vi "init.vi"(8 "error in (no error)":errorcluster, 11 "USD Actor in":refnum<class "USD Actor.lvclass">) -> (0 "error out":errorcluster, 3 "USD Actor out":refnum<class "USD Actor.lvclass">)   [LabVIEW 2020, in "USD Actor.lvlib" / "USD Actor.lvclass"]
uses:
  USD Actor.lvclass
  USD Actor.lvclass/USD Actor.ctl
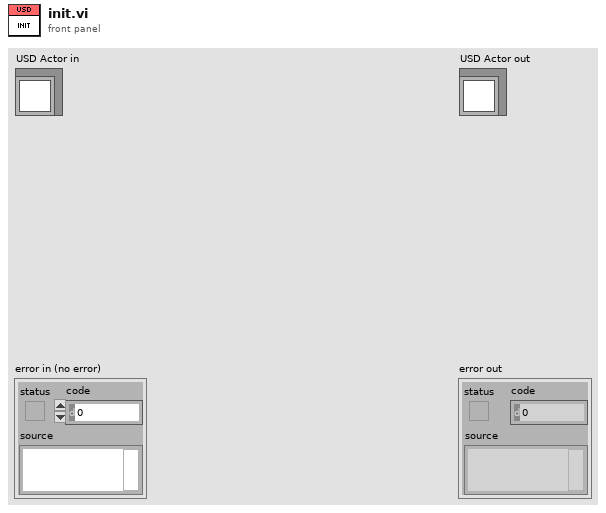
[diagram p1: front panel]
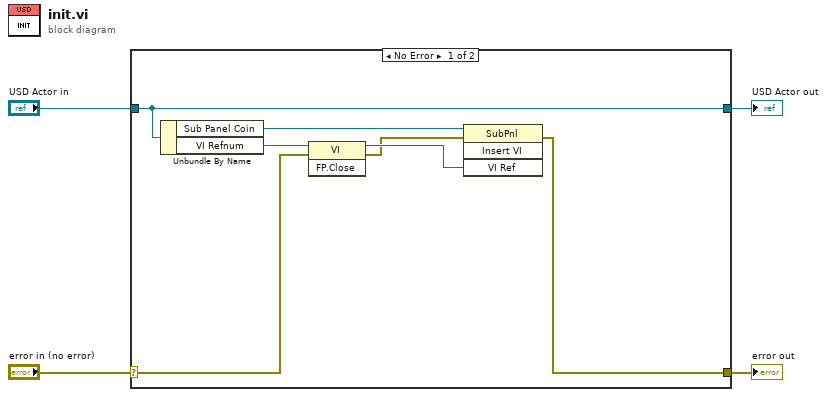
[diagram p0: block diagram]
diagram:
  n1 = case shown="No Error" "error in (no error)" {
    selector: "error in (no error)" -> [w7 w13]
    tunnel: [w6 w13] -> w3
    tunnel: [w11 w12] -> w1
    tunnel: "USD Actor in" -> [w11 w12]
    frame No Error {
      n2 = Unbundle By Name(w11) -> ("Sub Panel Coin"=w10:refnum<vi>, "VI Refnum"=w9:refnum<vi>)
      n3 = invoke class="VI" method="FP.Close"(reference=w9, error in=w7) -> (reference out=w8:refnum<vi>, error out=w5:errorcluster)  [unwired: 1 in, 1 out]
      n4 = invoke class="SubPnl" method="Insert VI"(reference=w10, error in=w5, "VI Ref"=w8) -> (error out=w6:errorcluster)  [unwired: 1 in, 3 out]
    }
    frame Error {
    }
  }
  "error out" <- w3
  "USD Actor out" <- w1
